vi "Is Value a number.vi"(8 "user error in":errorcluster, 11 "value String":string) -> (0 "user error out":errorcluster, 1 "number":dbl, 2 "a number":bool, 3 "value String out":string)   [LabVIEW 2011]
panel:
  out "error message 2":string
  in  "error message in":string
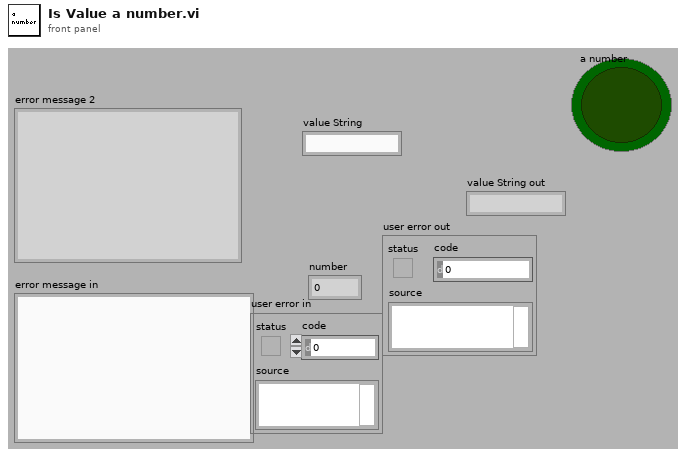
[diagram p1: front panel]
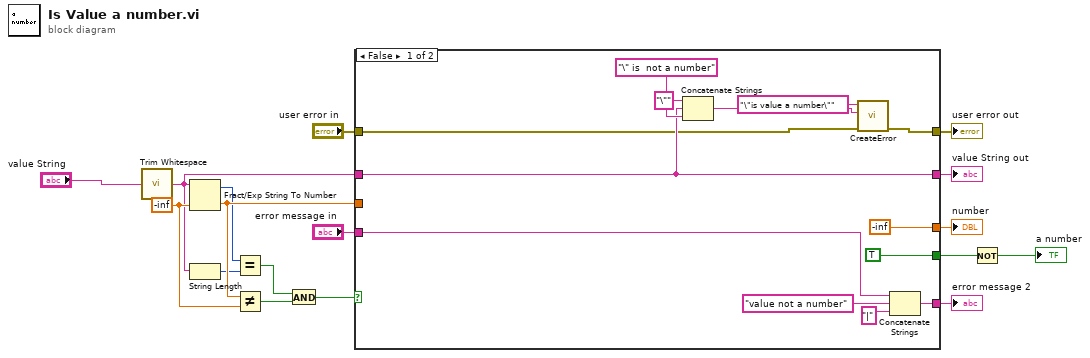
[diagram p0: block diagram]
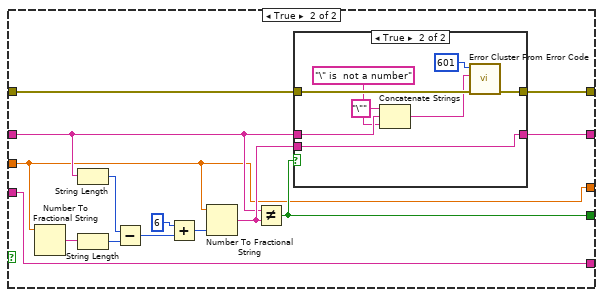
[diagram p2: hidden frame]
diagram:
  w17 = -inf
  n1 = call "Trim Whitespace.vi"("string"="value String") -> ("trimmed string"=w12:string)  [unwired: 1 in]
  n2 = Fract/Exp String To Number(string=w12, default (0 dbl)=w17) -> (offset past number=w11:i32, number=w15:dbl)  [unwired: 2 in]
  n3 = String Length(string=w12) -> (length=w10:i32)
  n4 = Equal?(x=w11, y=w10) -> (x = y?=w9:bool)
  n5 = Not Equal?(x=w15, y=w17) -> (x != y?=w8:bool)
  n6 = And(x=w9, y=w8) -> (x .and. y?=w7:bool)
  n7 = case shown="False" w7 {
    tunnel: "error message in" -> [w28 w39]
    tunnel: [w27 w39] -> w13
    tunnel: w15 -> [_ w31]
    tunnel: w12 -> [w22 w32]
    tunnel: [w22 w33] -> w14
    tunnel: [TRUE w37] -> w6
    tunnel: "user error in" -> [w21 w36]
    tunnel: [w20 w35] -> w4
    tunnel: [-inf w31] -> w2
    frame False {
      n8 = Concatenate Strings("\"" ("string"), w22, "\" is  not a number") -> (w19:string)
      n9 = call "CreateError.vi"("user error in"=w21, "error message (\"\")"=w19, "command"="\"is value a number\"") -> ("user error  out"=w20:errorcluster)  [unwired: 8 in]
      n10 = Concatenate Strings(w28, "value not a number", "|") -> (w27:string)
    }
    frame True {
      n11 = Number To Fractional String(number=w31) -> (F-format string=w44:string)  [unwired: 3 in]
      n12 = String Length(string=w32) -> (length=w40:i32)
      n13 = String Length(string=w44) -> (length=w43:i32)
      n14 = Subtract(x=w40, y=w43) -> (x-y=w42:i32)
      n15 = Add(x=6, y=w42) -> (x+y=w38:i32)
      n16 = Number To Fractional String(number=w31, precision (6)=w38) -> (F-format string=w34:string)  [unwired: 2 in]
      n17 = Not Equal?(x=w32, y=w34) -> (x != y?=w37:bool)
      n18 = case shown="True" w37 {
        tunnel: w36 -> [w46 w53]
        tunnel: [w46 w52] -> w35
        tunnel: w34 -> [_ w51]
        tunnel: [w45 w51] -> w33
        tunnel: w32 -> [w45 w50]
        frame False {
        }
        frame True {
          n19 = Concatenate Strings("\"" ("string"), w50, "\" is  not a number") -> (w47:string)
          n20 = call <vilib>:"Error Cluster From Error Code.vi"("error in (no error)"=w53, "error message (\"\")"=w47, "error code (0)"=601) -> ("error out"=w52:errorcluster)  [unwired: 6 in]
        }
      }
    }
  }
  "value String out" <- w14
  "error message 2" <- w13
  "user error out" <- w4
  "number" <- w2
  n21 = Not(x=w6) -> (.not. x?=→"a number":bool)
